vi "_Parse Markdown Doc Elements.vi"(8 "Error in":errorcluster caption="Error in (no error)", 11 "Lines":string[](array[string])) -> (0 "Error out":errorcluster, 2 "Array":T1[](array[typedef]), 3 "Lines (dup)":string[](array[string]))   [LabVIEW 2017, in "csmdoc.lvlib"]
uses:
  csmdoc.lvlib
  _Typedef/DocElement.ctl
  _tool/_file/csm-file-support.lvlib
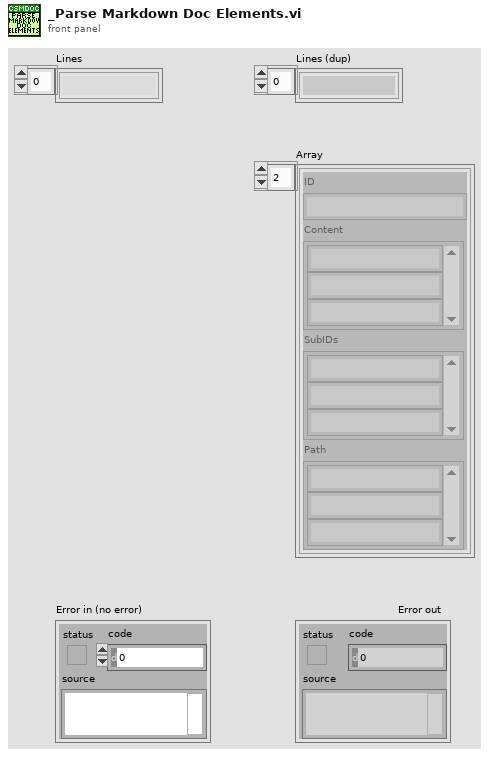
[diagram p1: front panel]
types:
  T1 = typedef "csmdoc.lvlib/DocElement.ctl" = cluster{"ID":string, "Content":string[], "SubIDs":string[], "Path":string[]}
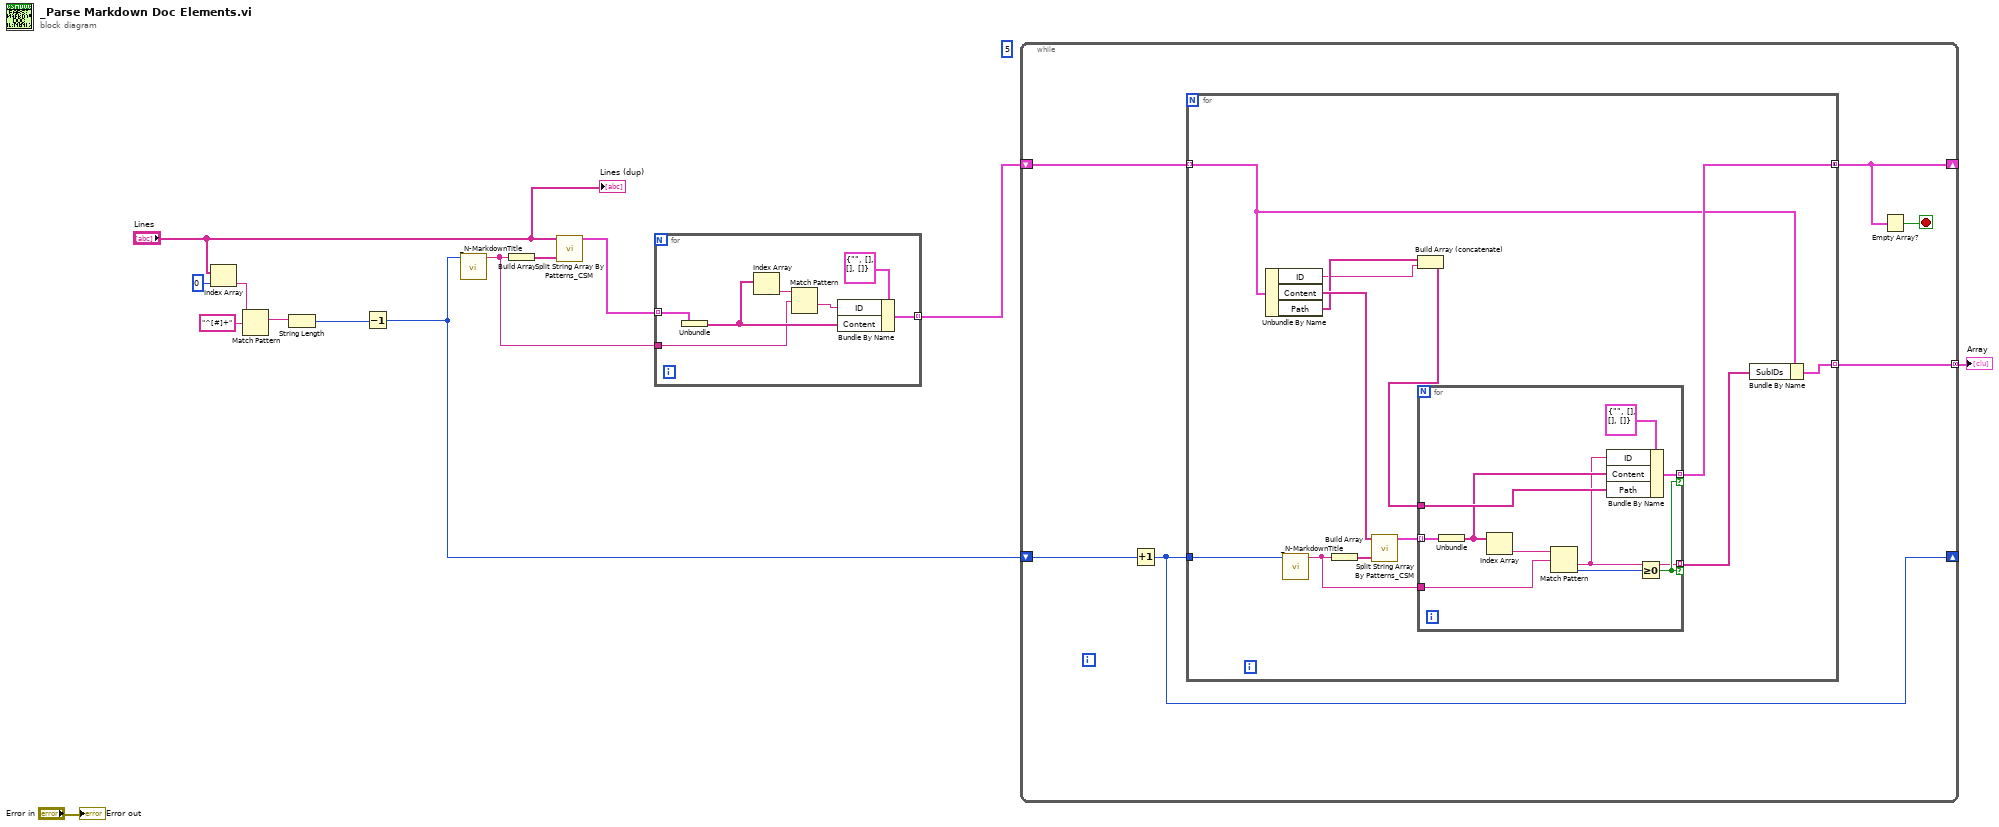
[diagram p0: block diagram]
diagram:
  (unwired) 5
  n1 = Index Array(array="Lines", index=0) -> (element=w5:string)
  n2 = Match Pattern(string=w5, regular expression="^[#]+") -> (match substring=w3:string)  [unwired: 1 in, 3 out]
  n3 = String Length(string=w3) -> (length=w2:i32)
  n4 = Decrement(x=w2) -> (x-1=w1:i32)
  n5 = call "_N-MarkdownTitle.vi"("Numeric"=w1) -> ("String"=w12:string)  [unwired: 10 in]
  n6 = Build Array(w12) -> (w9:string[])
  n7 = call "Split String Array By Patterns_CSM.vi"("Patterns"=w9, "Text Array"="Lines") -> ("Array"=w10:cluster{"filtered array":string[]}[])  [unwired: 9 in]
  n8 = for {
    tunnel: w10 -> [w19] mode=indexing
    tunnel: [w15] -> w11 mode=indexing
    tunnel: w12 -> [w14]
    n9 = Unbundle(w19) -> ("filtered array"=w16:string[])
    n10 = Index Array(array=w16) -> (element=w18:string)  [unwired: 1 in]
    n11 = Match Pattern(string=w18, regular expression=w14) -> (after substring=w17:string)  [unwired: 1 in, 3 out]
    n12 = Bundle By Name(cluster=T1 {"ID"="", "Content"=[], "SubIDs"=[], "Path"=[]} ("Cluster"), "ID"=w17, "Content"=w16) -> (w15:T1)
  }
  n13 = while {
    shift-right: [w23] -> _
    shift-left: w11 -> [w26]
    tunnel: [w25] -> w13 mode=concatenating
    shift-right: [w21] -> _
    shift-left: w1 -> [w22]
    stop <- w24 stop-if-true
    n14 = Increment(x=w22) -> (x+1=w21:i32)
    n15 = for {
      tunnel: w26 -> [w27] mode=indexing
      tunnel: w21 -> [w36]
      tunnel: [w34] -> w25 mode=indexing
      tunnel: [w29] -> w23 mode=concatenating
      n16 = Unbundle By Name(w27) -> ("ID"=w31:string, "Content"=w33:string[], "Path"=w32:string[])
      n17 = call "_N-MarkdownTitle.vi"("Numeric"=w36) -> ("String"=w28:string)  [unwired: 10 in]
      n18 = Build Array(w28) -> (w38:string[])
      n19 = call "Split String Array By Patterns_CSM.vi"("Patterns"=w38, "Text Array"=w33) -> ("Array"=w37:cluster{"filtered array":string[]}[])  [unwired: 9 in]
      n20 = Build Array (concatenate)(w32, w31) -> (w30:string[])
      n21 = for {
        tunnel: w37 -> [w48] mode=indexing
        tunnel: w28 -> [w47]
        tunnel: [w39] -> w35 mode=indexing if=w40
        tunnel: w30 -> [w44]
        tunnel: [w41] -> w29 mode=indexing if=w40
        n22 = Unbundle(w48) -> ("filtered array"=w43:string[])
        n23 = Index Array(array=w43) -> (element=w42:string)  [unwired: 1 in]
        n24 = Match Pattern(string=w42, regular expression=w47) -> (after substring=w39:string, offset past match=w46:i32)  [unwired: 1 in, 2 out]
        n25 = Bundle By Name(cluster=T1 {"ID"="", "Content"=[], "SubIDs"=[], "Path"=[]} ("Cluster"), "ID"=w39, "Content"=w43, "Path"=w44) -> (w41:T1)
        n26 = Greater Or Equal To 0?(x=w46) -> (x >= 0?=w40:bool)
      }
      n27 = Bundle By Name(cluster=w27, "SubIDs"=w35) -> (w34:T1)
    }
    n28 = Empty Array?(array=w23) -> (empty?=w24:bool)
  }
  "Array" <- w13
  "Lines (dup)" <- "Lines"
  "Error out" <- "Error in"
